vi "Load Sequence.vi"(6 "Fallback Name":string, 7 "CRC":u32 format="%08x", 8 "error in (no error)":refnum<class "MultiErrors.lvclass">, 10 "Config Element":refnum<class "Config Element.lvclass">) -> (0 "error out":refnum<class "MultiErrors.lvclass">, 3 "Sequence Config out":refnum<class "Sequence Config.lvclass">)   [LabVIEW 2023, in "VolatusSeqConfig.lvlib" / "Sequence Config.lvclass"]
uses:
  Sequence Config.lvclass
  VolatusErrorUtilities/MultiErrors/MultiErrors.lvclass
  lv-cdm/CDM-Config/Config Element/Config Element.lvclass
  Debug Flags.ctl
  VolatusErrorUtilities/MultiErrors/MultiErrors.lvclass/MultiErrors.ctl
  Sequence Config.lvclass/Sequence Config.ctl
  Sequence Constants/Sequence Constants.lvclass
  VolatusSeqConfig.lvlib
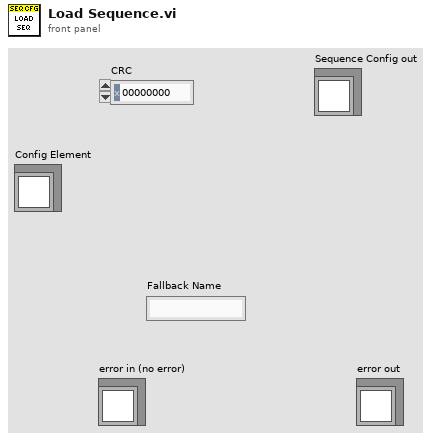
[diagram p1: front panel]
types:
  T1 = typedef "VolatusSeqConfig.lvlib/Debug Flags.ctl" = cluster{"States":bool, "Conditions":bool, "Timing":bool}
  T2 = typedef "VolatusSeqConfig.lvlib/Variable.ctl" = cluster{"Name":string, "Value":dbl, "Comment":string}
  T3 = typedef "VolatusSeqConfig.lvlib/State.ctl" = cluster{"Name":string, "Steps":T4[], "Transitions":refnum<class "Transition Config.lvclass">[], "Comment":string, "Color":string, "Seq Name":string, "Debug":T1}
  T4 = typedef "VolatusSeqConfig.lvlib/Step.ctl" = cluster{"Time":dbl, "Commands":refnum<class "Command Config.lvclass">[]}
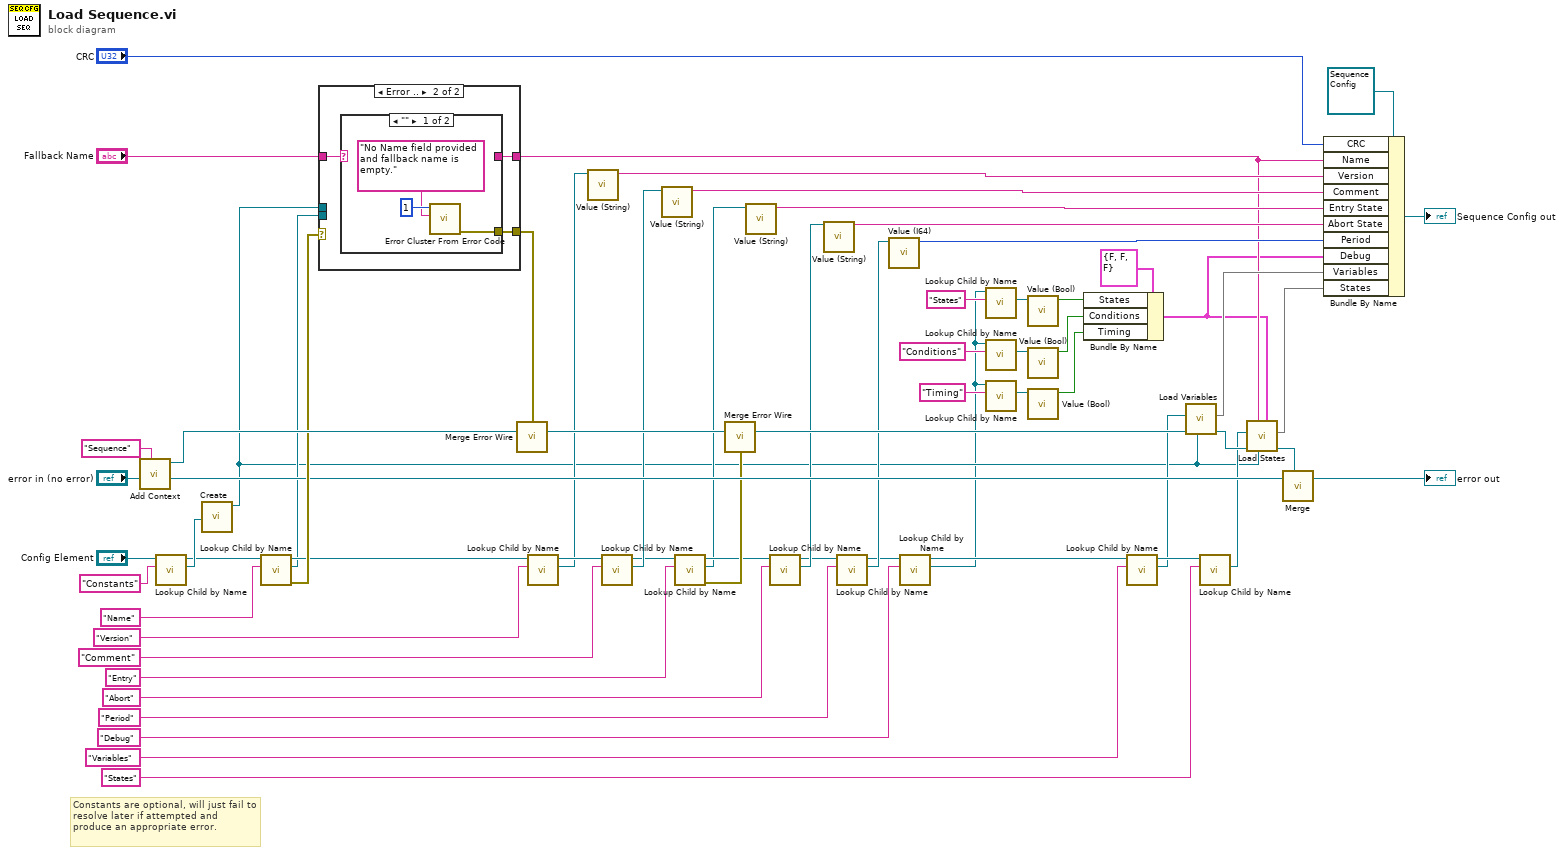
[diagram p0: block diagram]
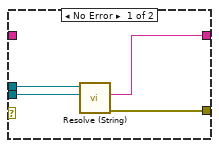
[diagram p2: hidden frame]
diagram:
  # "Constants are optional, will just fail to resolve later if attempted and produce an appropriate error."
  n1 = call "Add Context.vi"("Context"="Sequence", "MultiErrors in"="error in (no error)") -> ("Original Context"=w63:refnum<class "MultiErrors.lvclass">, "Added Context"=w66:refnum<class "MultiErrors.lvclass">)  [unwired: 8 in]
  n2 = call "Lookup Child by Name.vi"("Name"="Constants", "Config Element in"="Config Element") -> ("Child"=w22:refnum<class "Config Element.lvclass">, "Config Element out"=w10:refnum<class "Config Element.lvclass">)  [unwired: 6 in, 2 out]
  n3 = call "Create.vi"("Element"=w22) -> ("Sequence Constants out"=w9:refnum<class "Sequence Constants.lvclass">)  [unwired: 9 in, 1 out]
  n4 = call "Lookup Child by Name.vi"("Name"="Name", "Config Element in"=w10) -> ("error out"=w64:errorcluster, "Child"=w32:refnum<class "Config Element.lvclass">, "Config Element out"=w57:refnum<class "Config Element.lvclass">)  [unwired: 6 in, 1 out]
  n5 = case shown="Error .." w64 {
    tunnel: w32 -> [w70 _]
    tunnel: [w69 w72] -> w13
    tunnel: w9 -> [w68 _]
    tunnel: "Fallback Name" -> [_ w73]
    tunnel: [w67 w71] -> w6
    frame No Error {
      n6 = call "Resolve (String).vi"("Element"=w70, "Sequence Constants in"=w68) -> ("error out"=w67:errorcluster, "String Value"=w69:string)  [unwired: 7 in, 1 out]
    }
    frame Error {
      n7 = case shown="\"\"" w73 {
        selector: w73 -> [_ w77]
        tunnel: [_ w77] -> w72
        tunnel: [w74 _] -> w71
        frame "" {
          n8 = call <vilib>:"Error Cluster From Error Code.vi"("error message (\"\")"="No Name field provided and fallback name is empty.", "error code (0)"=1) -> ("error out"=w74:errorcluster)  [unwired: 7 in]
        }
        frame Default {
        }
      }
    }
  }
  n9 = call "Merge Error Wire.vi"("error in (no error)"=w6, "MultiErrors in"=w66) -> ("MultiErrors out"=w65:refnum<class "MultiErrors.lvclass">)  [unwired: 13 in]
  n10 = call "Lookup Child by Name.vi"("Name"="Version", "Config Element in"=w57) -> ("Child"=w48:refnum<class "Config Element.lvclass">, "Config Element out"=w55:refnum<class "Config Element.lvclass">)  [unwired: 6 in, 2 out]
  n11 = call "Value (String).vi"("Config Element in"=w48) -> ("String Value"=w47:string)  [unwired: 9 in, 1 out]
  n12 = call "Lookup Child by Name.vi"("Name"="Comment", "Config Element in"=w55) -> ("Child"=w46:refnum<class "Config Element.lvclass">, "Config Element out"=w34:refnum<class "Config Element.lvclass">)  [unwired: 6 in, 2 out]
  n13 = call "Value (String).vi"("Config Element in"=w46) -> ("String Value"=w45:string)  [unwired: 9 in, 1 out]
  n14 = call "Lookup Child by Name.vi"("Name"="Entry", "Config Element in"=w34) -> ("error out"=w62:errorcluster, "Child"=w39:refnum<class "Config Element.lvclass">, "Config Element out"=w40:refnum<class "Config Element.lvclass">)  [unwired: 6 in, 1 out]
  n15 = call "Merge Error Wire.vi"("error in (no error)"=w62, "MultiErrors in"=w65) -> ("MultiErrors out"=w61:refnum<class "MultiErrors.lvclass">)  [unwired: 13 in]
  n16 = call "Value (String).vi"("Config Element in"=w39) -> ("String Value"=w36:string)  [unwired: 9 in, 1 out]
  n17 = call "Lookup Child by Name.vi"("Name"="Abort", "Config Element in"=w40) -> ("Child"=w37:refnum<class "Config Element.lvclass">, "Config Element out"=w27:refnum<class "Config Element.lvclass">)  [unwired: 6 in, 2 out]
  n18 = call "Value (String).vi"("Config Element in"=w37) -> ("String Value"=w35:string)  [unwired: 9 in, 1 out]
  n19 = call "Lookup Child by Name.vi"("Name"="Period", "Config Element in"=w27) -> ("Child"=w24:refnum<class "Config Element.lvclass">, "Config Element out"=w21:refnum<class "Config Element.lvclass">)  [unwired: 6 in, 2 out]
  n20 = call "Value (I64).vi"("Config Element in"=w24) -> ("I64 Value"=w25:i64)  [unwired: 9 in, 1 out]
  n21 = call "Lookup Child by Name.vi"("Name"="Debug", "Config Element in"=w21) -> ("Child"=w3:refnum<class "Config Element.lvclass">, "Config Element out"=w8:refnum<class "Config Element.lvclass">)  [unwired: 6 in, 2 out]
  n22 = call "Lookup Child by Name.vi"("Name"="States", "Config Element in"=w3) -> ("Child"=w16:refnum<class "Config Element.lvclass">)  [unwired: 6 in, 3 out]
  n23 = call "Lookup Child by Name.vi"("Name"="Conditions", "Config Element in"=w3) -> ("Child"=w14:refnum<class "Config Element.lvclass">)  [unwired: 6 in, 3 out]
  n24 = call "Lookup Child by Name.vi"("Name"="Timing", "Config Element in"=w3) -> ("Child"=w5:refnum<class "Config Element.lvclass">)  [unwired: 6 in, 3 out]
  n25 = call "Value (Bool).vi"("Config Element in"=w16) -> ("Bool Value"=w15:bool)  [unwired: 9 in, 1 out]
  n26 = call "Value (Bool).vi"("Config Element in"=w14) -> ("Bool Value"=w12:bool)  [unwired: 9 in, 1 out]
  n27 = call "Value (Bool).vi"("Config Element in"=w5) -> ("Bool Value"=w2:bool)  [unwired: 9 in, 1 out]
  n28 = Bundle By Name(cluster=T1 {"States"=FALSE, "Conditions"=FALSE, "Timing"=FALSE} ("Events"), "States"=w15, "Conditions"=w12, "Timing"=w2) -> (w1:T1)
  n29 = call "Lookup Child by Name.vi"("Name"="Variables", "Config Element in"=w8) -> ("Child"=w50:refnum<class "Config Element.lvclass">, "Config Element out"=w52:refnum<class "Config Element.lvclass">)  [unwired: 6 in, 2 out]
  n30 = call "Load Variables.vi"("Constants"=w9, "error in (no error)"=w61, "Config Element"=w50) -> ("error out"=w60:refnum<class "MultiErrors.lvclass">, "Variables"=w44:map{string, T2})  [unwired: 7 in]
  n31 = call "Lookup Child by Name.vi"("Name"="States", "Config Element in"=w52) -> ("Child"=w43:refnum<class "Config Element.lvclass">)  [unwired: 6 in, 3 out]
  n32 = call "Load States.vi"("Debug"=w1, "Constants"=w9, "Seq Name"=w13, "error in"=w60, "Config Element"=w43) -> ("error out"=w29:refnum<class "MultiErrors.lvclass">, "States"=w42:map{string, T3})  [unwired: 5 in]
  n33 = call "Merge.vi"("First Error In"=w63, "Second Error In"=w29) -> ("MultiErrors out"=→"error out":refnum<class "MultiErrors.lvclass">)  [unwired: 5 in]
  n34 = Bundle By Name(cluster=refnum<class "Sequence Config.lvclass"> refnum ("Sequence Config in"), "CRC"="CRC", "Name"=w13, "Version"=w47, "Comment"=w45, "Entry State"=w36, "Abort State"=w35, "Period"=w25, "Debug"=w1, "Variables"=w44, "States"=w42) -> (→"Sequence Config out":refnum<class "Sequence Config.lvclass">)
